vi "RecordinsideStep.vi"(6 "More_Info":string, 8 "error in (no error)":errorcluster, 9 "STEP":string, 10 "Station":string, 11 "SN":string) -> (0 "error out":errorcluster)   [LabVIEW 2020]
uses:
  <vilib>/Utility/config.llb/Read Key (String).vi
  <vilib>/Utility/config.llb/Write Key (String).vi
  <vilib>/Utility/config.llb/NI_LVConfig.lvlib
panel:
  out "appended path":path
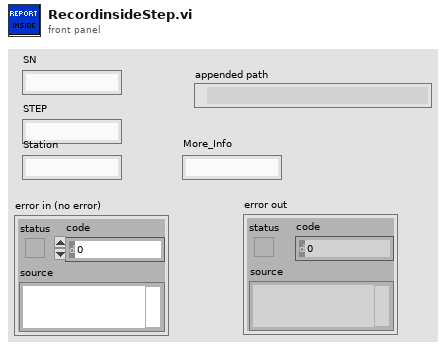
[diagram p1: front panel]
types:
  T1 = typedef "NI_LVConfig.lvlib/Config Data RefNum.ctl" = refnum<k1>
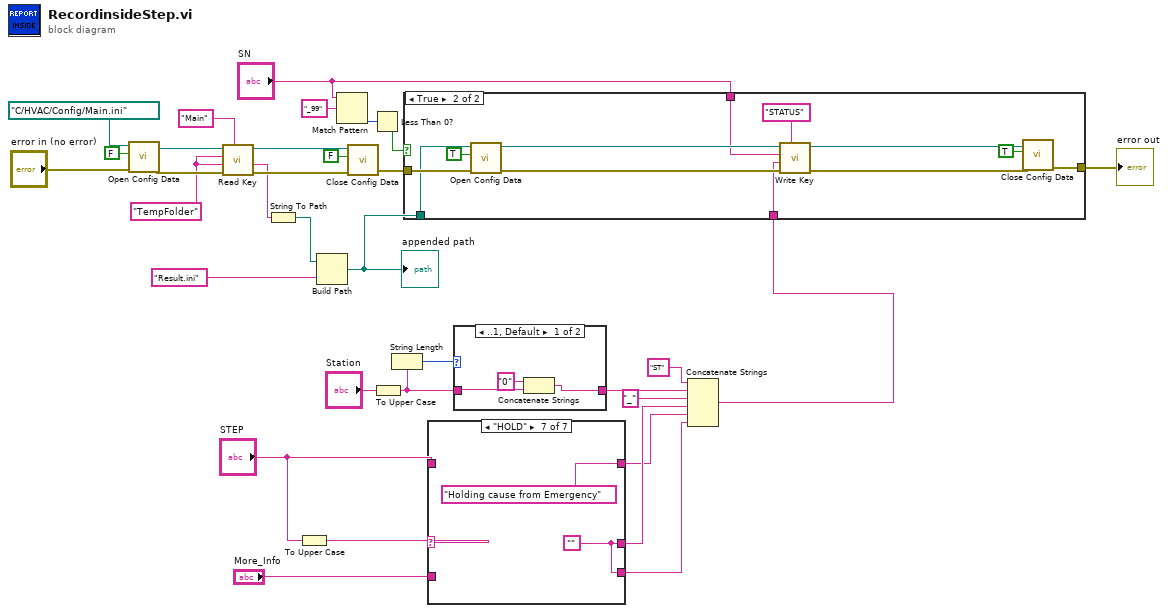
[diagram p0: block diagram]
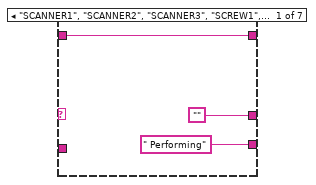
[diagram p4: hidden frame]
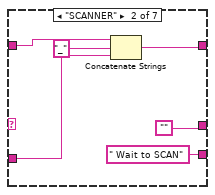
[diagram p5: hidden frame]
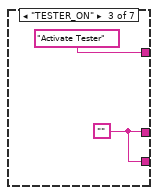
[diagram p6: hidden frame]
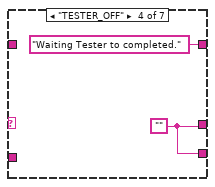
[diagram p7: hidden frame]
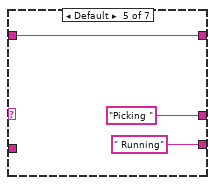
[diagram p8: hidden frame]
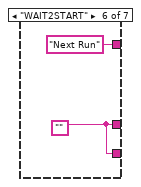
[diagram p9: hidden frame]
diagram:
  w30 = "TempFolder" ("key")
  n1 = call <vilib>:"Open Config Data.vi"("error in (no error)"="error in (no error)", "create file if necessary (T)"=FALSE, "configuration file path"=path "C:/HVAC/Config/Main.ini") -> ("error out"=w32:errorcluster, "refnum"=w31:T1)  [unwired: 6 in, 1 out]
  n2 = call-poly <vilib>:"Read Key.vi"("section"="Main", "error in (no error)"=w32, "default value"=w30, "key"=w30, "refnum"=w31) -> ("error out"=w28:errorcluster, "value"=w25:string, "refnum out"=w27:T1)  [unwired: 3 in, 1 out]
  n3 = String To Path(string=w25) -> (path=w20:path)
  n4 = To Upper Case(1:"STEP") -> (0:w12:string)
  n5 = Build Path(base path=w20, name or relative path="Result.ini" ("time format string (%c)")) -> (appended path=w23:path)
  "appended path" <- w23
  n6 = Match Pattern(string="SN", regular expression="_99") -> (offset past match=w3:i32)  [unwired: 1 in, 3 out]
  n7 = call <vilib>:"Close Config Data.vi"("error in (no error)"=w28, "write file if changed (T)"=FALSE, "refnum"=w27) -> ("error out"=w24:errorcluster)  [unwired: 7 in, 1 out]
  n8 = Less Than 0?(x=w3) -> (x < 0?=w2:bool)
  n9 = To Upper Case(1:"Station") -> (0:w7:string)
  n10 = String Length(string=w7) -> (length=w6:i32)
  n11 = case shown="\"HOLD\"" w12 {
    tunnel: ["" "" w44 w46 "Picking " w50 w52] -> w13
    tunnel: [" Performing" ("string") " Wait to SCAN" ("string") w44 w46 " Running" ("string") w50 w52] -> w11
    tunnel: [w34 w40 "Activate Tester" "Waiting Tester to completed." ("STEP") w47 "Next Run" ("STEP") "Holding cause from Emergency" ("STEP")] -> w10
    tunnel: "STEP" -> [w34 w39 _ _ w47 _ _]
    tunnel: "More_Info" -> [_ w38 _ _ _ _ _]
    frame "SCANNER1", "SCANNER2", "SCANNER3", "SCREW1", "SCREW2" {
    }
    frame "SCANNER" {
      n12 = Concatenate Strings(w39, "_", w38) -> (w40:string)
    }
    frame "TESTER_ON" {
      w44 = ""
    }
    frame "TESTER_OFF" {
      w46 = ""
    }
    frame Default {
    }
    frame "WAIT2START" {
      w50 = ""
    }
    frame "HOLD" {
      w52 = ""
    }
  }
  n13 = case shown="..1, Default" w6 {
    tunnel: [w56 w57] -> w8
    tunnel: w7 -> [w55 w57]
    frame ..1, Default {
      n14 = Concatenate Strings("0" ("string"), w55) -> (w56:string)
    }
    frame 2.. {
    }
  }
  n15 = Concatenate Strings("ST", w8, "_" ("string"), w13, w10, w11) -> (w17:string)
  n16 = case shown="True" w2 {
    tunnel: w24 -> [w58 w70]
    tunnel: w23 -> [_ w69]
    tunnel: [w58 w62] -> w18
    tunnel: w17 -> [_ w60]
    tunnel: "SN" -> [_ w59]
    frame False {
    }
    frame True {
      n17 = call <vilib>:"Open Config Data.vi"("error in (no error)"=w70, "create file if necessary (T)"=TRUE, "configuration file path"=w69) -> ("error out"=w67:errorcluster, "refnum"=w66:T1)  [unwired: 6 in, 1 out]
      n18 = call-poly <vilib>:"Write Key.vi"("section"="STATUS", "error in (no error)"=w67, "value"=w60, "key"=w59, "refnum"=w66) -> ("error out"=w65:errorcluster, "refnum out"=w64:T1)  [unwired: 4 in, 1 out]
      n19 = call <vilib>:"Close Config Data.vi"("error in (no error)"=w65, "write file if changed (T)"=TRUE, "refnum"=w64) -> ("error out"=w62:errorcluster)  [unwired: 7 in, 1 out]
    }
  }
  "error out" <- w18
